vi "Pub-Sub Example.vi"   [LabVIEW 2024]
uses:
  NATS Infrastructure/NATS Infrastructure.lvlib
panel:
  # "Instructions:\n\n1. Run this VI\n2. Subscribe to a subject with Subscriber.vi\n3. Publish a message to the same subject with Publisher.vi\n4. Read with Subscriber.vi"
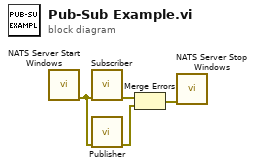
[diagram p0: block diagram]
diagram:
  n1 = call "NATS Server Start Windows.vi"() -> ("error out"=w3:errorcluster)  [unwired: 11 in]
  n2 = call "Subscriber.vi"("error in"=w3) -> ("error out"=w1:errorcluster)  [unwired: 10 in]
  n3 = call "Publisher.vi"("error in"=w3) -> ("error out"=w4:errorcluster)  [unwired: 10 in]
  n4 = Merge Errors(w1, w4) -> (w2:errorcluster)
  n5 = call "NATS Server Stop Windows.vi"("error in"=w2) -> ()  [unwired: 10 in, 1 out]
